vi "Eric's Project Greedy Snake simplified.vi"() -> ()   [LabVIEW 2020]
uses:
  <vilib>/event_ctls.llb/eventvkey.ctl
panel:
  out "String":string
  out "direction store":enum16{"left", "right", "up", "down"}(ring)=enum."right"
  in  "stop":bool
  in  "food?":bool=TRUE
  out "food location":i8[](array[numeric])
  out "snake coordinates":i8[][](array[numeric])
  out "VKey":T1
  in  "start/end game":bool
  in  "Difficulty":enum16{"low", "midium", "high"}(ring)=enum."high"
  in  "direction":enum16{"left", "right", "up", "down"}(ring)=enum."right"
  in  "Boundary Height":i8=15 min=5 max=15
  in  "Boundary Width":i8=15 min=5 max=15
  out "map":bool[][](array[boolean])
  # "maximun 15*15"
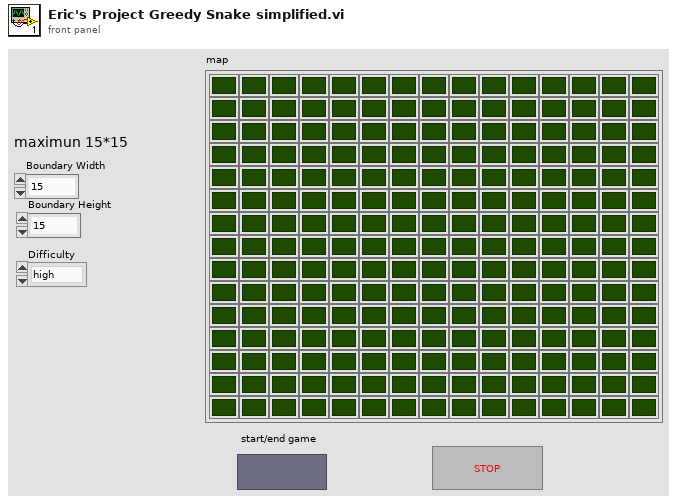
[diagram p1: front panel]
types:
  T1 = typedef "eventvkey.ctl" = enum16{"ASCII", "Enter", "Return", "Shift", "Ctrl", "Alt", "Cmd", "Opt", "Caps", "NumLock", "Clear", "Break", "Up", "Down", "Left", "Right", "Insert", "Delete", "Home", "End", "PageUp", "PageDown", "Escape", "Help", "Pause", "ScrollLock", "F1", "F2", "F3", "F4", "F5", "F6", "F7", "F8", "F9", "F10", "F11", "F12", "F13", "F14", "F15", "F16", "F17", "F18", "F19", "F20", "F21", "F22", "F23", "F24", "Play", "VolumeUp", "VolumeDown", "Mute", "Two Byte Char"}
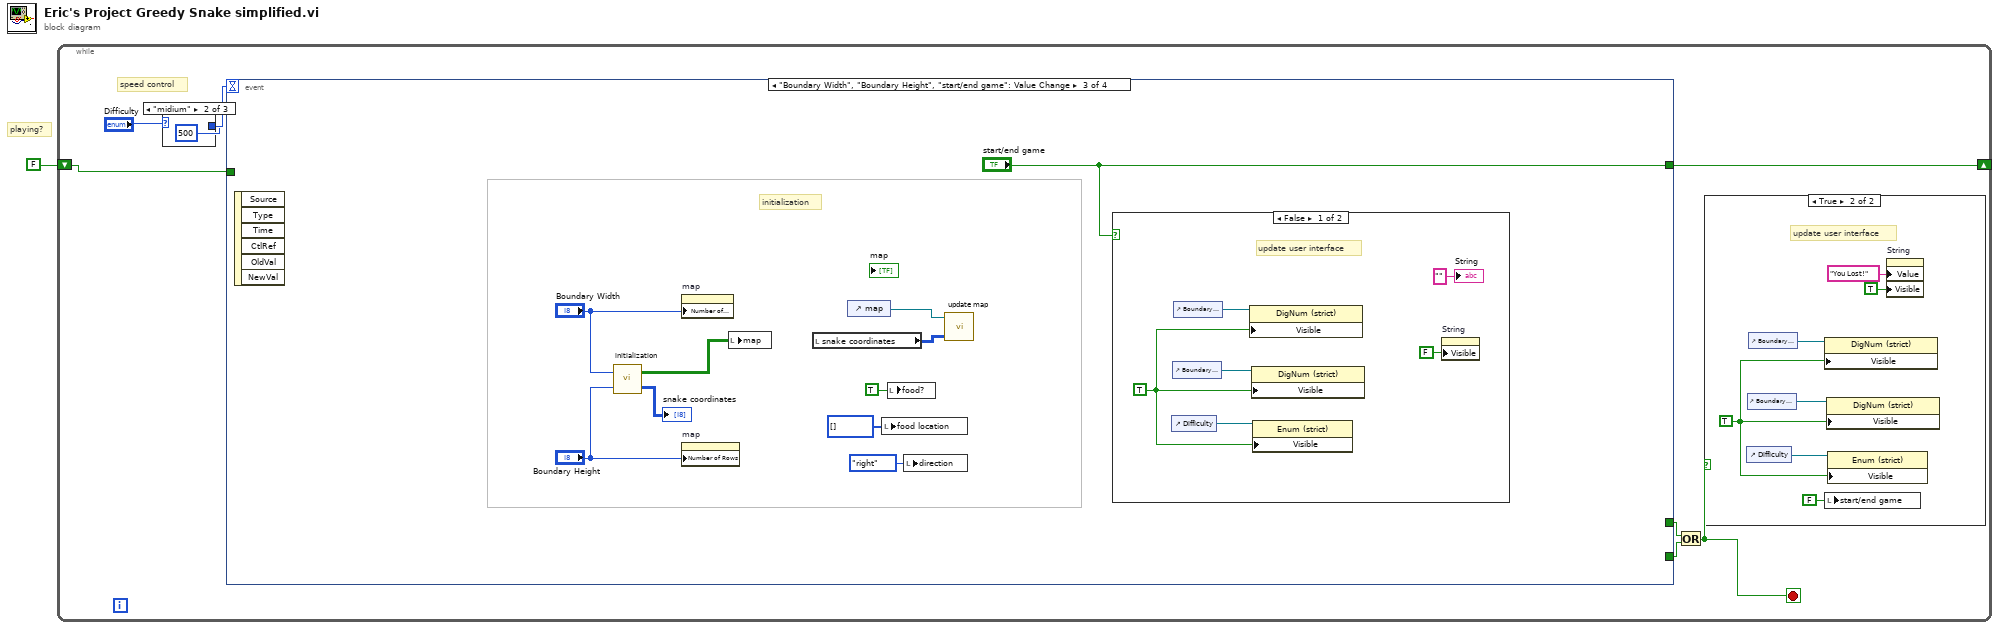
[diagram p0: block diagram]
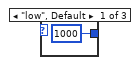
[diagram p3: hidden frame]
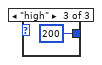
[diagram p4: hidden frame]
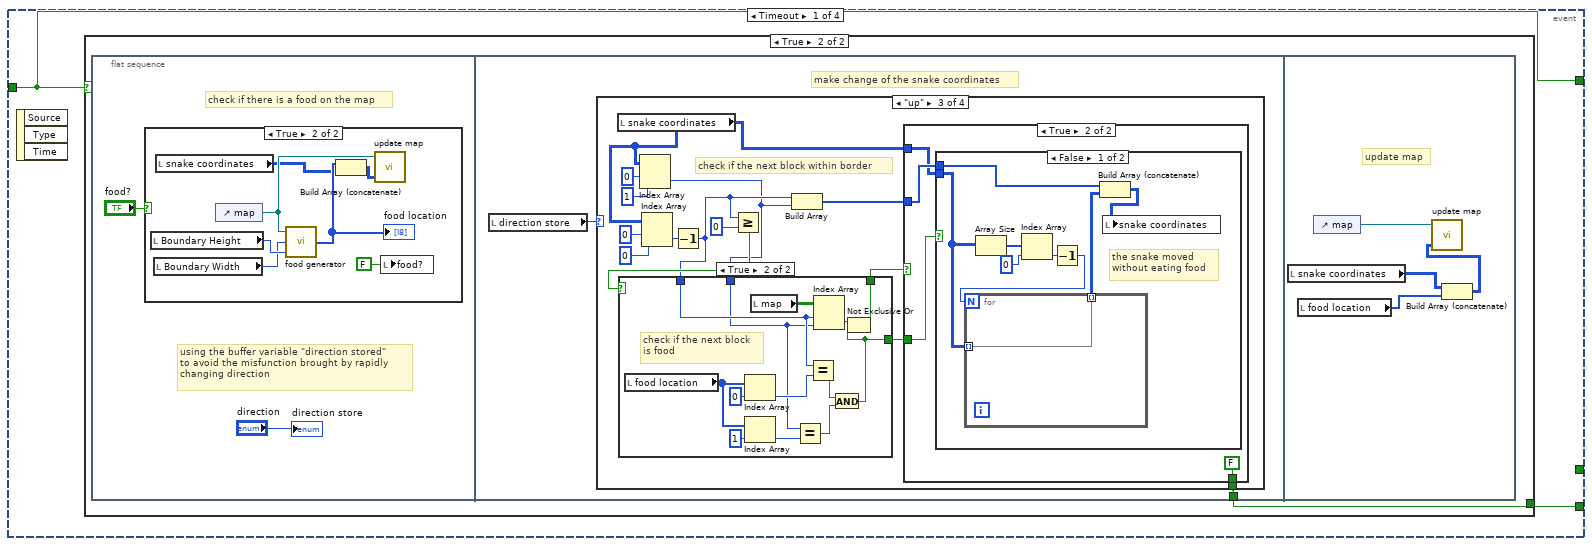
[diagram p5: hidden frame]
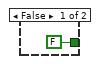
[diagram p6: hidden frame]
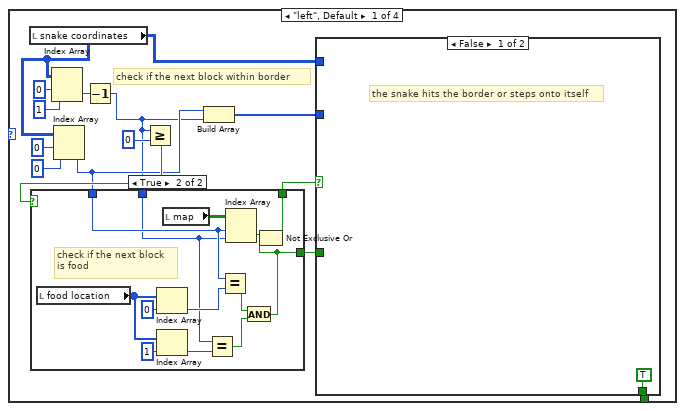
[diagram p8: hidden frame]
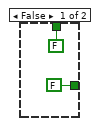
[diagram p9: hidden frame]
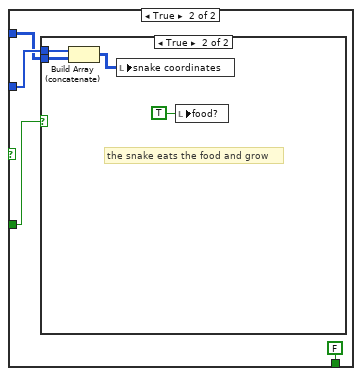
[diagram p10: hidden frame]
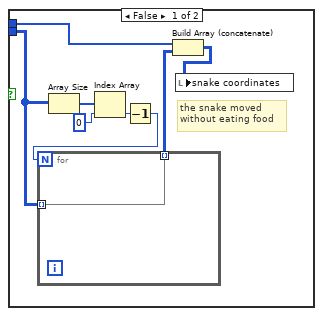
[diagram p11: hidden frame]
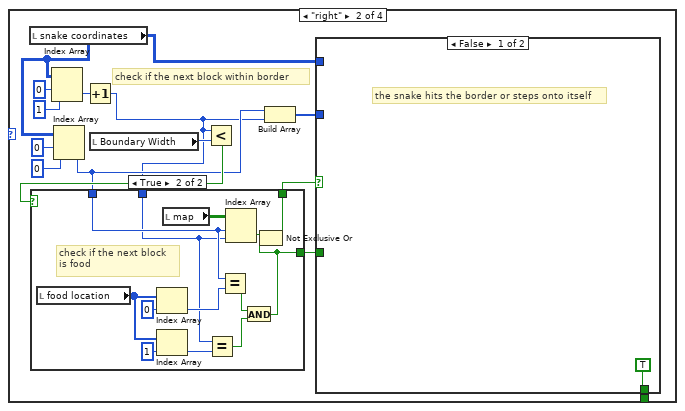
[diagram p12: hidden frame]
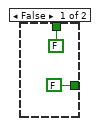
[diagram p13: hidden frame]
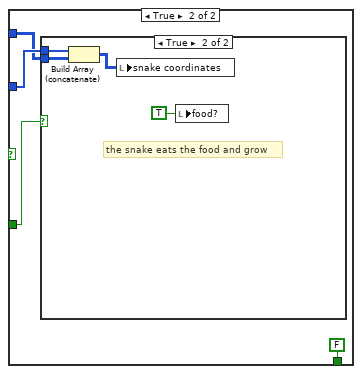
[diagram p14: hidden frame]
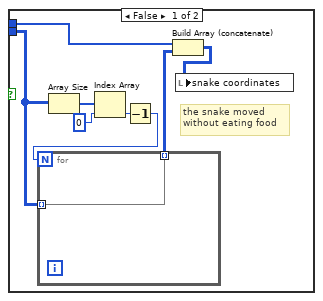
[diagram p15: hidden frame]
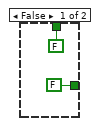
[diagram p16: hidden frame]
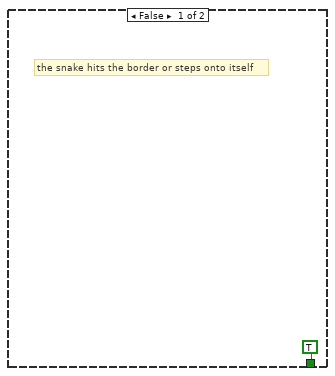
[diagram p17: hidden frame]
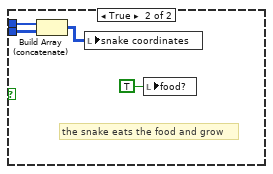
[diagram p18: hidden frame]
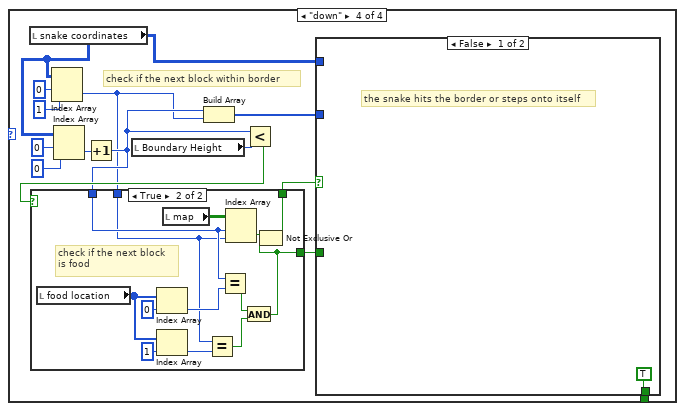
[diagram p19: hidden frame]
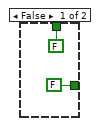
[diagram p20: hidden frame]
diagram:
  # "playing?"
  n1 = while {
    shift-right: [w7] -> _
    shift-left: FALSE -> [w3]
    stop <- w2 stop-if-true
    # "speed control"
    n2 = case shown="\"midium\"" "Difficulty" {
      tunnel: [u32 1000 ("milliseconds to wait") u32 500 ("milliseconds to wait") u32 200 ("milliseconds to wait")] -> w8
      frame "low", Default {
      }
      frame "midium" {
      }
      frame "high" {
      }
    }
    n3 = event shown="[2] \"Boundary Width\", \"Boundary Height\", \"start/end game\": Value Change" {
      selector: _ -> [_ _ _ _]
      dyn-events: _ -> [_ _ _ _]
      timeout: w8 -> [_ _ _ _]
      tunnel: [w20 _ _ _] -> w4
      tunnel: [_ _ _ "stop"] -> w5
      tunnel: [w19 w226 "start/end game" _] -> w7
      tunnel: w3 -> [w19 w226 _ _]
      event Timeout {
        n4 = event-data() -> ()  [unwired: 1 in, 3 out]
        n5 = case shown="True" w19 {
          tunnel: [FALSE w22] -> w20
          frame False {
          }
          frame True {
            n6 = flat-sequence {
              tunnel: [w33] -> w22
              frame #0 {
                # "using the buffer variable \"direction stored\"\nto avoid the misfunction brought by rapidly\nchanging direction"
                # "check if there is a food on the map"
                n7 = case shown="True" "food?" {
                  frame False {
                  }
                  frame True {
                    n8 = local read "Boundary Height"() -> (w31:i8)
                    n9 = local read "Boundary Width"() -> (w30:i8)
                    n10 = local read "snake coordinates"() -> (w25:i8[][])
                    n11 = control-ref of="map"() -> (w27:refnum<vi>)
                    n12 = call "food generator.vi"("Boundary Height"=w31, "Boundary Width"=w30, "Array in"=w27) -> ("food location"=w29:i8[])
                    "food location" <- w29
                    n13 = Build Array (concatenate)(w29, w25) -> (w28:i8[][])
                    n14 = call "update map.vi"("coordinates"=w28, "Array in"=w27) -> ()  [unwired: 1 in]
                    n15 = local write "food?"(FALSE ("food?")) -> ()
                  }
                }
                "direction store" <- "direction"
              }
              frame #1 {
                # "make change of the snake coordinates"
                n16 = local read "direction store"() -> (w32:enum16{"left", "right", "up", "down"})
                n17 = case shown="\"up\"" w32 {
                  tunnel: [w38 w86 w133 w181] -> w33
                  frame "left", Default {
                    # "check if the next block within border"
                    n18 = local read "snake coordinates"() -> (w37:i8[][])
                    n19 = Index Array(array=w37, index (row)=0, index (col)=1 ("disabled index (col)")) -> (element=w45:i8)
                    n20 = Index Array(array=w37, index (row)=0, index (col)=0 ("disabled index (col)")) -> (element=w36:i8)
                    n21 = Decrement(x=w45) -> (x-1=w35:i8)
                    n22 = Greater Or Equal?(x=w35, y=i8 0) -> (x >= y?=w40:bool)
                    n23 = case shown="True" w40 {
                      tunnel: [FALSE w51] -> w39
                      tunnel: w36 -> [_ w59]
                      tunnel: w35 -> [_ w55]
                      tunnel: [FALSE w50] -> w42
                      frame False {
                      }
                      frame True {
                        # "check if the next block\nis food"
                        n24 = local read "food location"() -> (w57:i8[])
                        n25 = Index Array(array=w57, index=0) -> (element=w60:i8)
                        n26 = Index Array(array=w57, index=1) -> (element=w56:i8)
                        n27 = local read "map"() -> (w62:bool[][])
                        n28 = Equal?(x=w55, y=w56) -> (x = y?=w53:bool)
                        n29 = Equal?(x=w59, y=w60) -> (x = y?=w54:bool)
                        n30 = Index Array(array=w62, index (row)=w59, index (col)=w55) -> (element=w52:bool)
                        n31 = And(x=w54, y=w53) -> (x .and. y?=w50:bool)
                        n32 = Not Exclusive Or(1:w50, 2:w52) -> (0:w51:bool)
                      }
                    }
                    n33 = Build Array(w36, w35) -> (w34:i8[])
                    n34 = case shown="False" w39 {
                      tunnel: w42 -> [_ w64]
                      tunnel: [TRUE FALSE] -> w38
                      tunnel: w37 -> [_ w65]
                      tunnel: w34 -> [_ w66]
                      frame False {
                        # "the snake hits the border or steps onto itself"
                      }
                      frame True {
                        n35 = case shown="True" w64 {
                          tunnel: w66 -> [w70 w80]
                          tunnel: w65 -> [w75 w79]
                          frame False {
                            # "the snake moved \nwithout eating food"
                            n36 = Array Size(array=w75) -> (size(s)=w74:i32[])
                            n37 = Index Array(array=w74, index=0) -> (element=w72:i32)
                            n38 = Decrement(x=w72) -> (x-1=w71:i32)
                            n39 = for {
                              N: w71 -> [_]
                              tunnel: w75 -> [w76] mode=indexing
                              tunnel: [w76] -> w69 mode=indexing
                            }
                            n40 = Build Array (concatenate)(w70, w69) -> (w68:i8[][])
                            n41 = local write "snake coordinates"(w68) -> ()
                          }
                          frame True {
                            # "the snake eats the food and grow"
                            n42 = Build Array (concatenate)(w80, w79) -> (w77:i8[][])
                            n43 = local write "snake coordinates"(w77) -> ()
                            n44 = local write "food?"(TRUE ("food?")) -> ()
                          }
                        }
                      }
                    }
                  }
                  frame "right" {
                    # "check if the next block within border"
                    n45 = local read "snake coordinates"() -> (w85:i8[][])
                    n46 = Index Array(array=w85, index (row)=0, index (col)=1 ("disabled index (col)")) -> (element=w92:i8)
                    n47 = Index Array(array=w85, index (row)=0, index (col)=0 ("disabled index (col)")) -> (element=w84:i8)
                    n48 = Increment(x=w92) -> (x+1=w81:i8)
                    n49 = local read "Boundary Width"() -> (w82:i8)
                    n50 = Less?(x=w81, y=w82) -> (x < y?=w88:bool)
                    n51 = case shown="True" w88 {
                      tunnel: [FALSE w98] -> w87
                      tunnel: w84 -> [_ w106]
                      tunnel: w81 -> [_ w102]
                      tunnel: [FALSE w97] -> w89
                      frame False {
                      }
                      frame True {
                        # "check if the next block\nis food"
                        n52 = local read "food location"() -> (w104:i8[])
                        n53 = Index Array(array=w104, index=0) -> (element=w107:i8)
                        n54 = Index Array(array=w104, index=1) -> (element=w103:i8)
                        n55 = local read "map"() -> (w109:bool[][])
                        n56 = Equal?(x=w102, y=w103) -> (x = y?=w100:bool)
                        n57 = Equal?(x=w106, y=w107) -> (x = y?=w101:bool)
                        n58 = Index Array(array=w109, index (row)=w106, index (col)=w102) -> (element=w99:bool)
                        n59 = And(x=w101, y=w100) -> (x .and. y?=w97:bool)
                        n60 = Not Exclusive Or(1:w97, 2:w99) -> (0:w98:bool)
                      }
                    }
                    n61 = Build Array(w84, w81) -> (w83:i8[])
                    n62 = case shown="False" w87 {
                      tunnel: w89 -> [_ w112]
                      tunnel: [TRUE FALSE] -> w86
                      tunnel: w85 -> [_ w113]
                      tunnel: w83 -> [_ w114]
                      frame False {
                        # "the snake hits the border or steps onto itself"
                      }
                      frame True {
                        n63 = case shown="True" w112 {
                          tunnel: w114 -> [w117 w127]
                          tunnel: w113 -> [w122 w126]
                          frame False {
                            # "the snake moved \nwithout eating food"
                            n64 = Array Size(array=w122) -> (size(s)=w121:i32[])
                            n65 = Index Array(array=w121, index=0) -> (element=w119:i32)
                            n66 = Decrement(x=w119) -> (x-1=w118:i32)
                            n67 = for {
                              N: w118 -> [_]
                              tunnel: w122 -> [w123] mode=indexing
                              tunnel: [w123] -> w116 mode=indexing
                            }
                            n68 = Build Array (concatenate)(w117, w116) -> (w115:i8[][])
                            n69 = local write "snake coordinates"(w115) -> ()
                          }
                          frame True {
                            # "the snake eats the food and grow"
                            n70 = Build Array (concatenate)(w127, w126) -> (w124:i8[][])
                            n71 = local write "snake coordinates"(w124) -> ()
                            n72 = local write "food?"(TRUE ("food?")) -> ()
                          }
                        }
                      }
                    }
                  }
                  frame "up" {
                    # "check if the next block within border"
                    n73 = local read "snake coordinates"() -> (w132:i8[][])
                    n74 = Index Array(array=w132, index (row)=0, index (col)=1 ("disabled index (col)")) -> (element=w128:i8)
                    n75 = Index Array(array=w132, index (row)=0, index (col)=0 ("disabled index (col)")) -> (element=w130:i8)
                    n76 = Decrement(x=w130) -> (x-1=w129:i8)
                    n77 = Greater Or Equal?(x=w129, y=i8 0) -> (x >= y?=w135:bool)
                    n78 = case shown="True" w135 {
                      tunnel: [FALSE w145] -> w134
                      tunnel: w129 -> [_ w153]
                      tunnel: w128 -> [_ w149]
                      tunnel: [FALSE w144] -> w137
                      frame False {
                      }
                      frame True {
                        # "check if the next block\nis food"
                        n79 = local read "food location"() -> (w151:i8[])
                        n80 = Index Array(array=w151, index=0) -> (element=w154:i8)
                        n81 = Index Array(array=w151, index=1) -> (element=w150:i8)
                        n82 = local read "map"() -> (w156:bool[][])
                        n83 = Equal?(x=w149, y=w150) -> (x = y?=w147:bool)
                        n84 = Equal?(x=w153, y=w154) -> (x = y?=w148:bool)
                        n85 = Index Array(array=w156, index (row)=w153, index (col)=w149) -> (element=w146:bool)
                        n86 = And(x=w148, y=w147) -> (x .and. y?=w144:bool)
                        n87 = Not Exclusive Or(1:w144, 2:w146) -> (0:w145:bool)
                      }
                    }
                    n88 = Build Array(w129, w128) -> (w131:i8[])
                    n89 = case shown="True" w134 {
                      tunnel: w137 -> [_ w158]
                      tunnel: [TRUE FALSE] -> w133
                      tunnel: w132 -> [_ w159]
                      tunnel: w131 -> [_ w160]
                      frame False {
                        # "the snake hits the border or steps onto itself"
                      }
                      frame True {
                        n90 = case shown="False" w158 {
                          tunnel: w160 -> [w164 w174]
                          tunnel: w159 -> [w169 w173]
                          frame False {
                            # "the snake moved \nwithout eating food"
                            n91 = Array Size(array=w169) -> (size(s)=w168:i32[])
                            n92 = Index Array(array=w168, index=0) -> (element=w166:i32)
                            n93 = Decrement(x=w166) -> (x-1=w165:i32)
                            n94 = for {
                              N: w165 -> [_]
                              tunnel: w169 -> [w170] mode=indexing
                              tunnel: [w170] -> w163 mode=indexing
                            }
                            n95 = Build Array (concatenate)(w164, w163) -> (w162:i8[][])
                            n96 = local write "snake coordinates"(w162) -> ()
                          }
                          frame True {
                            # "the snake eats the food and grow"
                            n97 = Build Array (concatenate)(w174, w173) -> (w171:i8[][])
                            n98 = local write "snake coordinates"(w171) -> ()
                            n99 = local write "food?"(TRUE ("food?")) -> ()
                          }
                        }
                      }
                    }
                  }
                  frame "down" {
                    # "check if the next block within border"
                    n100 = local read "snake coordinates"() -> (w180:i8[][])
                    n101 = Index Array(array=w180, index (row)=0, index (col)=1 ("disabled index (col)")) -> (element=w175:i8)
                    n102 = Index Array(array=w180, index (row)=0, index (col)=0 ("disabled index (col)")) -> (element=w178:i8)
                    n103 = Increment(x=w178) -> (x+1=w176:i8)
                    n104 = local read "Boundary Height"() -> (w177:i8)
                    n105 = Build Array(w176, w175) -> (w179:i8[])
                    n106 = Less?(x=w176, y=w177) -> (x < y?=w183:bool)
                    n107 = case shown="True" w183 {
                      tunnel: [FALSE w192] -> w182
                      tunnel: w176 -> [_ w200]
                      tunnel: w175 -> [_ w196]
                      tunnel: [FALSE w191] -> w184
                      frame False {
                      }
                      frame True {
                        # "check if the next block\nis food"
                        n108 = local read "food location"() -> (w198:i8[])
                        n109 = Index Array(array=w198, index=0) -> (element=w201:i8)
                        n110 = Index Array(array=w198, index=1) -> (element=w197:i8)
                        n111 = local read "map"() -> (w203:bool[][])
                        n112 = Equal?(x=w196, y=w197) -> (x = y?=w194:bool)
                        n113 = Equal?(x=w200, y=w201) -> (x = y?=w195:bool)
                        n114 = Index Array(array=w203, index (row)=w200, index (col)=w196) -> (element=w193:bool)
                        n115 = And(x=w195, y=w194) -> (x .and. y?=w191:bool)
                        n116 = Not Exclusive Or(1:w191, 2:w193) -> (0:w192:bool)
                      }
                    }
                    n117 = case shown="False" w182 {
                      tunnel: w184 -> [_ w205]
                      tunnel: [TRUE FALSE] -> w181
                      tunnel: w180 -> [_ w206]
                      tunnel: w179 -> [_ w207]
                      frame False {
                        # "the snake hits the border or steps onto itself"
                      }
                      frame True {
                        n118 = case shown="True" w205 {
                          tunnel: w207 -> [w211 w221]
                          tunnel: w206 -> [w216 w220]
                          frame False {
                            # "the snake moved \nwithout eating food"
                            n119 = Array Size(array=w216) -> (size(s)=w215:i32[])
                            n120 = Index Array(array=w215, index=0) -> (element=w213:i32)
                            n121 = Decrement(x=w213) -> (x-1=w212:i32)
                            n122 = for {
                              N: w212 -> [_]
                              tunnel: w216 -> [w217] mode=indexing
                              tunnel: [w217] -> w210 mode=indexing
                            }
                            n123 = Build Array (concatenate)(w211, w210) -> (w209:i8[][])
                            n124 = local write "snake coordinates"(w209) -> ()
                          }
                          frame True {
                            # "the snake eats the food and grow"
                            n125 = Build Array (concatenate)(w221, w220) -> (w218:i8[][])
                            n126 = local write "snake coordinates"(w218) -> ()
                            n127 = local write "food?"(TRUE ("food?")) -> ()
                          }
                        }
                      }
                    }
                  }
                }
              }
              frame #2 {
                # "update map"
                n128 = local read "snake coordinates"() -> (w223:i8[][])
                n129 = local read "food location"() -> (w224:i8[])
                n130 = control-ref of="map"() -> (w222:refnum<vi>)
                n131 = Build Array (concatenate)(w223, w224) -> (w225:i8[][])
                n132 = call "update map.vi"("coordinates"=w225, "Array in"=w222) -> ()  [unwired: 1 in]
              }
            }
          }
        }
      }
      event Key Down {
        # "the buffer variable prevents the user\nfrom changing to an illegal direction\nthat may end the game(say from left to right)"
        # "change direction of the snakes movement"
        n133 = event-data() -> ("VKey"=→"VKey":T1)  [unwired: 1 in, 9 out]
        n134 = local read "direction store"() -> (w230:enum16{"left", "right", "up", "down"})
        n135 = local read "VKey"() -> (w227:T1)
        n136 = case shown="\"up\"" w230 {
          tunnel: w227 -> [w232 w237 w242 w247]
          tunnel: [w231 w236 w241 w246] -> w229
          frame "left", Default {
            n137 = case shown="\"Insert\", Default" w232 {
              tunnel: [w233 enum16{"left", "right", "up", "down"}."up" ("direction") enum16{"left", "right", "up", "down"}."down" ("direction")] -> w231
              frame "Insert", Default {
                n138 = local read "direction store"() -> (w233:enum16{"left", "right", "up", "down"})
              }
              frame "Up" {
              }
              frame "Down" {
              }
            }
          }
          frame "right" {
            n139 = case shown="\"Insert\", Default" w237 {
              tunnel: [w238 enum16{"left", "right", "up", "down"}."up" ("direction") enum16{"left", "right", "up", "down"}."down" ("direction")] -> w236
              frame "Insert", Default {
                n140 = local read "direction store"() -> (w238:enum16{"left", "right", "up", "down"})
              }
              frame "Up" {
              }
              frame "Down" {
              }
            }
          }
          frame "up" {
            n141 = case shown="\"Left\"" w242 {
              tunnel: [w243 enum16{"left", "right", "up", "down"}."left" ("direction") enum16{"left", "right", "up", "down"}."right" ("direction")] -> w241
              frame "Insert", Default {
                n142 = local read "direction store"() -> (w243:enum16{"left", "right", "up", "down"})
              }
              frame "Left" {
              }
              frame "Right" {
              }
            }
          }
          frame "down" {
            n143 = case shown="\"Insert\", Default" w247 {
              tunnel: [w248 enum16{"left", "right", "up", "down"}."left" ("direction") enum16{"left", "right", "up", "down"}."right" ("direction")] -> w246
              frame "Insert", Default {
                n144 = local read "direction store"() -> (w248:enum16{"left", "right", "up", "down"})
              }
              frame "Left" {
              }
              frame "Right" {
              }
            }
          }
        }
        n145 = local write "direction"(w229) -> ()
      }
      event "Boundary Width", "Boundary Height", "start/end game": Value Change {
        # "initialization"
        n146 = event-data() -> ()  [unwired: 1 in, 6 out]
        n147 = call "initialization.vi"("Boundary Height"="Boundary Height", "Boundary Width"="Boundary Width") -> ("snake coordinates"=→"snake coordinates":i8[][], "map"=w258:bool[][])
        n148 = property on="map" class="Arr (strict)"("Number of Columns"="Boundary Width") -> ()  [unwired: 2 in, 2 out]
        n149 = property on="map" class="Arr (strict)"("Number of Rows"="Boundary Height") -> ()  [unwired: 2 in, 2 out]
        n150 = local write "map"(w258) -> ()
        n151 = local read "snake coordinates"() -> (w255:i8[][])
        n152 = control-ref of="map"() -> (w254:refnum<vi>)
        n153 = local write "food location"(i8[] [] ("food location")) -> ()
        n154 = local write "food?"(TRUE ("food?")) -> ()
        n155 = local write "direction"(enum16{"left", "right", "up", "down"}."right" ("direction")) -> ()
        n156 = call "update map.vi"("coordinates"=w255, "Array in"=w254) -> ()  [unwired: 1 in]
        n157 = case shown="False" "start/end game" {
          frame False {
            w263 = TRUE ("Visible")
            # "update user interface"
            n158 = control-ref of="Difficulty"() -> (w264:refnum<vi>)
            n159 = control-ref of="Boundary Height"() -> (w265:refnum<vi>)
            n160 = control-ref of="Boundary Width"() -> (w266:refnum<vi>)
            n161 = property class="DigNum (strict)"(reference=w266, "Visible"=w263) -> ()  [unwired: 1 in, 2 out]
            n162 = property class="DigNum (strict)"(reference=w265, "Visible"=w263) -> ()  [unwired: 1 in, 2 out]
            n163 = property class="Enum (strict)"(reference=w264, "Visible"=w263) -> ()  [unwired: 1 in, 2 out]
            n164 = property on="String" class="Str"("Visible"=FALSE) -> ()  [unwired: 2 in, 2 out]
            "String" <- "" ("String")
          }
          frame True {
            w267 = FALSE ("Visible")
            # "update user interface"
            n165 = control-ref of="Difficulty"() -> (w268:refnum<vi>)
            n166 = control-ref of="Boundary Height"() -> (w269:refnum<vi>)
            n167 = control-ref of="Boundary Width"() -> (w270:refnum<vi>)
            n168 = property class="DigNum (strict)"(reference=w270, "Visible"=w267) -> ()  [unwired: 1 in, 2 out]
            n169 = property class="DigNum (strict)"(reference=w269, "Visible"=w267) -> ()  [unwired: 1 in, 2 out]
            n170 = property class="Enum (strict)"(reference=w268, "Visible"=w267) -> ()  [unwired: 1 in, 2 out]
          }
        }
      }
      event "stop": Value Change {
        n171 = event-data() -> ()  [unwired: 1 in, 6 out]
      }
    }
    n172 = Or(x=w5, y=w4) -> (x .or. y?=w2:bool)
    n173 = case shown="True" w2 {
      frame False {
      }
      frame True {
        w12 = TRUE ("Visible")
        # "update user interface"
        n174 = control-ref of="Difficulty"() -> (w15:refnum<vi>)
        n175 = control-ref of="Boundary Height"() -> (w14:refnum<vi>)
        n176 = control-ref of="Boundary Width"() -> (w13:refnum<vi>)
        n177 = property class="DigNum (strict)"(reference=w13, "Visible"=w12) -> ()  [unwired: 1 in, 2 out]
        n178 = local write "start/end game"(FALSE ("start/end game")) -> ()
        n179 = property class="DigNum (strict)"(reference=w14, "Visible"=w12) -> ()  [unwired: 1 in, 2 out]
        n180 = property class="Enum (strict)"(reference=w15, "Visible"=w12) -> ()  [unwired: 1 in, 2 out]
        n181 = property on="String" class="Str"("Value"="You Lost!" ("String"), "Visible"=TRUE) -> ()  [unwired: 2 in, 2 out]
      }
    }
  }
